vi "String math.vi"() -> ()   [LabVIEW 2020]
panel:
  out "SDO":u64[](array[numeric]) format="%.0x"
  out "max(x,y)":i32[](array[numeric])
  out "y":i32
  out "number":u64[](array[numeric]) format="%.0x"
  out "Array":string[](array[string])
  in  "String":string
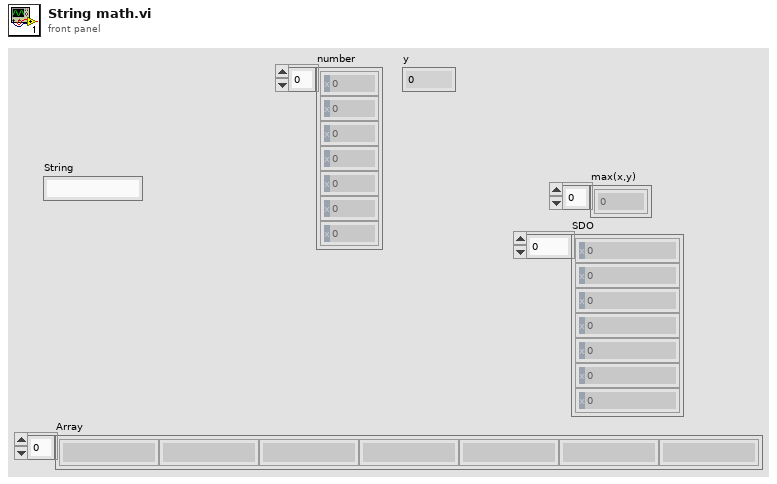
[diagram p1: front panel]
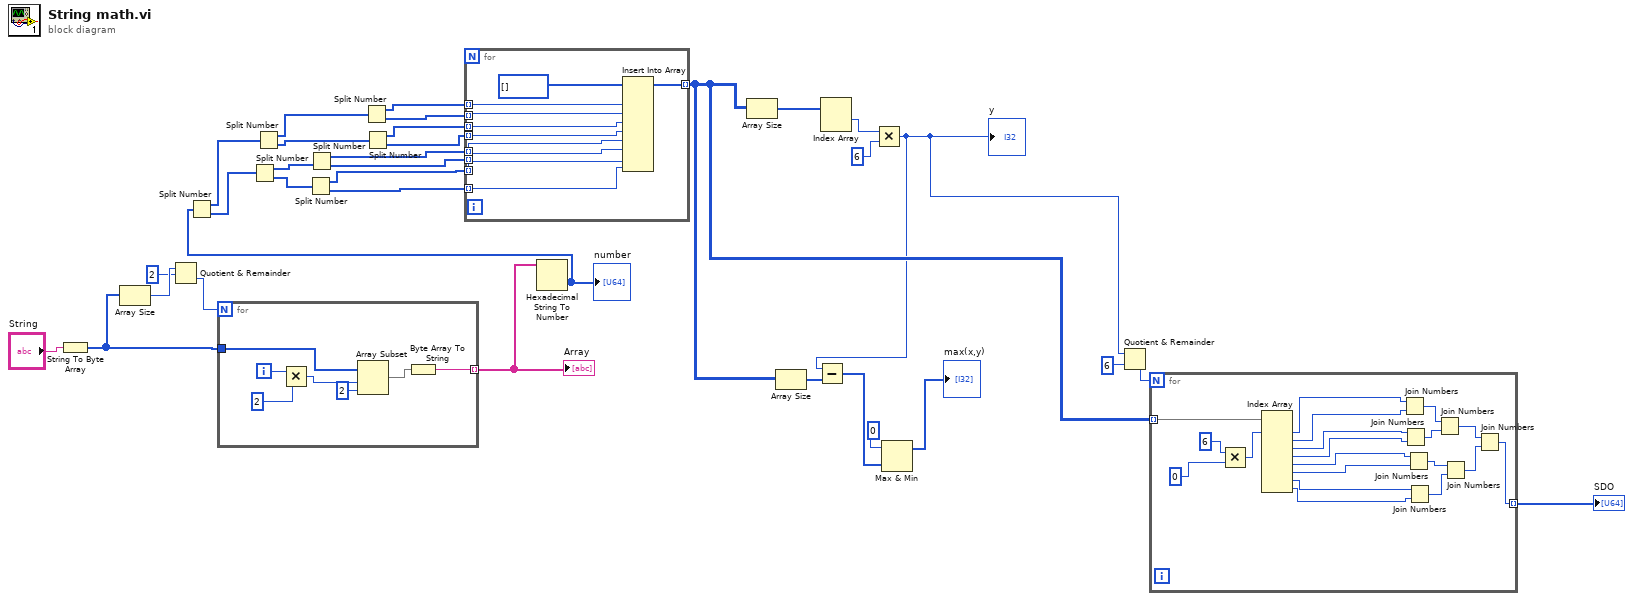
[diagram p0: block diagram]
diagram:
  n1 = String To Byte Array(string="String") -> (unsigned byte array=w32:u8[])
  n2 = Array Size(array=w32) -> (size(s)=w31:i32)
  n3 = Quotient & Remainder(x=w31, y=2) -> (floor(x/y)=w29:i32)  [unwired: 1 out]
  n4 = for {
    N: w29 -> [_]
    tunnel: w32 -> [w40]
    tunnel: [w35] -> w28 mode=indexing
    i -> [w39]
    n5 = Multiply(x=w39, y=2) -> (x*y=w37:i32)
    n6 = Array Subset(array=w40, index=w37, length=2) -> (w34:u8[])
    n7 = Byte Array To String(unsigned byte array=w34) -> (string=w35:string)
  }
  "Array" <- w28
  n8 = Hexadecimal String To Number(string=w28) -> (number=w13:u32[])  [unwired: 2 in, 1 out]
  "number" <- w13
  n9 = Split Number(x=w13) -> (hi(x)=w23:u16[], lo(x)=w24:u16[])
  n10 = Split Number(x=w24) -> (hi(x)=w25:u8[], lo(x)=w18:u8[])
  n11 = Split Number(x=w23) -> (hi(x)=w27:u8[], lo(x)=w26:u8[])
  n12 = Split Number(x=w18) -> (hi(x)=w15:u8[], lo(x)=w14:u8[])
  n13 = Split Number(x=w25) -> (hi(x)=w17:u8[], lo(x)=w16:u8[])
  n14 = Split Number(x=w27) -> (hi(x)=w22:u8[], lo(x)=w21:u8[])
  n15 = Split Number(x=w26) -> (hi(x)=w20:u8[], lo(x)=w19:u8[])
  n16 = for {
    tunnel: [w50] -> w2 mode=indexing
    tunnel: w22 -> [w48] mode=indexing
    tunnel: w21 -> [w47] mode=indexing
    tunnel: w20 -> [w46] mode=indexing
    tunnel: w19 -> [w45] mode=indexing
    tunnel: w17 -> [w44] mode=indexing
    tunnel: w16 -> [w43] mode=indexing
    tunnel: w15 -> [w42] mode=indexing
    tunnel: w14 -> [w41] mode=indexing
    n17 = Insert Into Array(array=u8[] [], new element #1=w48, new element #2=w47, new element #3=w46, new element #4=w45, new element #5=w44, new element #6=w43, new element #7=w42, new element #8=w41) -> (w50:u8[])  [unwired: 1 in]
  }
  n18 = Array Size(array=w2) -> (size(s)=w12:i32[])
  n19 = Array Size(array=w2) -> (size(s)=w6:i32[])
  n20 = Index Array(array=w12) -> (element #1=w11:i32)  [unwired: 2 in, 1 out]
  n21 = Multiply(x=w11, y=6) -> (x*y=w1:i32)
  "y" <- w1
  n22 = Subtract(x=w1, y=w6) -> (x-y=w9:i32[])
  n23 = Max & Min(x=0, y=w9) -> (max(x,y)=→"max(x,y)":i32[])  [unwired: 1 out]
  n24 = Quotient & Remainder(x=w1, y=6) -> (floor(x/y)=w4:i32)  [unwired: 1 out]
  n25 = for {
    N: w4 -> [_]
    tunnel: [w67] -> w3 mode=indexing
    tunnel: w2 -> [w66] mode=indexing
    n26 = Multiply(x=6, y=0) -> (x*y=w68:i32)
    n27 = Index Array(array=w66, index #1=w68) -> (element #1=w59:u8, element #2=w58:u8, element #3=w57:u8, element #4=w56:u8, element #5=w55:u8, element #6=w54:u8, element #7=w53:u8, element #8=w52:u8)  [unwired: 7 in]
    n28 = Join Numbers(hi=w59, lo=w58) -> ((hi.lo)=w61:u16)
    n29 = Join Numbers(hi=w57, lo=w56) -> ((hi.lo)=w60:u16)
    n30 = Join Numbers(hi=w55, lo=w54) -> ((hi.lo)=w63:u16)
    n31 = Join Numbers(hi=w53, lo=w52) -> ((hi.lo)=w62:u16)
    n32 = Join Numbers(hi=w61, lo=w60) -> ((hi.lo)=w65:u32)
    n33 = Join Numbers(hi=w63, lo=w62) -> ((hi.lo)=w64:u32)
    n34 = Join Numbers(hi=w65, lo=w64) -> ((hi.lo)=w67:u64)
  }
  "SDO" <- w3
